vi "run.vi"(8 "error in (no error)":errorcluster, 11 "DL090409StageScaffold in":refnum<class "StageDL090409Scaffold.lvclass">) -> (0 "error out":errorcluster, 3 "DL090409StageScaffold out":refnum<class "StageDL090409Scaffold.lvclass">)   [LabVIEW 2010, in "StageDL090409Scaffold.lvclass"]
uses:
  StageDL090409Scaffold.lvclass
  main/labview_source/controls/undock_button.ctl
  internal_trigger_enum.ctl
  state_enum.ctl
  common/classes/SpaceVector/SpaceVector/SpaceVector.lvclass
  StageDL090409Scaffold.lvclass/StageDL090409Scaffold.ctl
  common/enumerations/top-level_component_type_enum.ctl
  GenericStage/GenericStage/trigger_enum.ctl
  GenericStage/GenericStage/translation_mode_enum.ctl
  stored_data_cluster.ctl
  common/classes/Image/Image/Image.lvclass
  Display/GenericDisplay/GenericDisplay/GenericDisplay.lvclass
  common/classes/GenericToplevelComponent/GenericToplevelComponent/trigger_type_enum.ctl
  GenericStage/GenericStage/GenericStage.lvclass
  common/classes/GenericToplevelComponent/GenericToplevelComponent/GenericToplevelComponent.lvclass
  common/classes/ErrorController/ErrorController/class_data.vi
  common/classes/ErrorController/ErrorController/ErrorController.lvclass
panel:
  in  "Tab Control":enum32{"User", "Debug", "About"}(tab)
  out "current x":dbl[unit] caption="x"
  out "current y":dbl[unit] caption="y"
  out "current z":dbl[unit] caption="z"
  in  "setOriginButton":bool
  in  "step x":dbl[unit] caption="x"
  in  "step y":dbl[unit] caption="y"
  in  "step z":dbl[unit] caption="z"
  in  "stepButton":bool
  in  "returnToOriginButton":bool
  in  "Stored positions":i32(listbox)
  in  "Description":string
  in  "store button":bool
  out "position image":T1(plugin-control)
  in  "go to stored button":bool
  in  "remove stored item":bool
  in  "step x 2":dbl[unit] caption="x"
  in  "step y 2":dbl[unit] caption="y"
  in  "step z 2":dbl[unit] caption="z"
  in  "moveAbsolute":bool
  in  "button:undock":T2
  out "finished?":bool
  out "last trigger":T3=enum."initialise"
  out "state":T4
  out "statemachine loop counter":i32
  out "event loop error":errorcluster
  out "statemachine error":errorcluster
  out "event loop counter":i32
  # "Move"
  # "Current position"
  # "Move To:"
  # "Make sure that\nALL axes have correct values!!!"
  # "StageDL090409Scaffold (or child class)\n\nimplemented by: Dominik Langer, University of Zurich\nmodified by: Marcel van 't Hoff, University of Zurich"
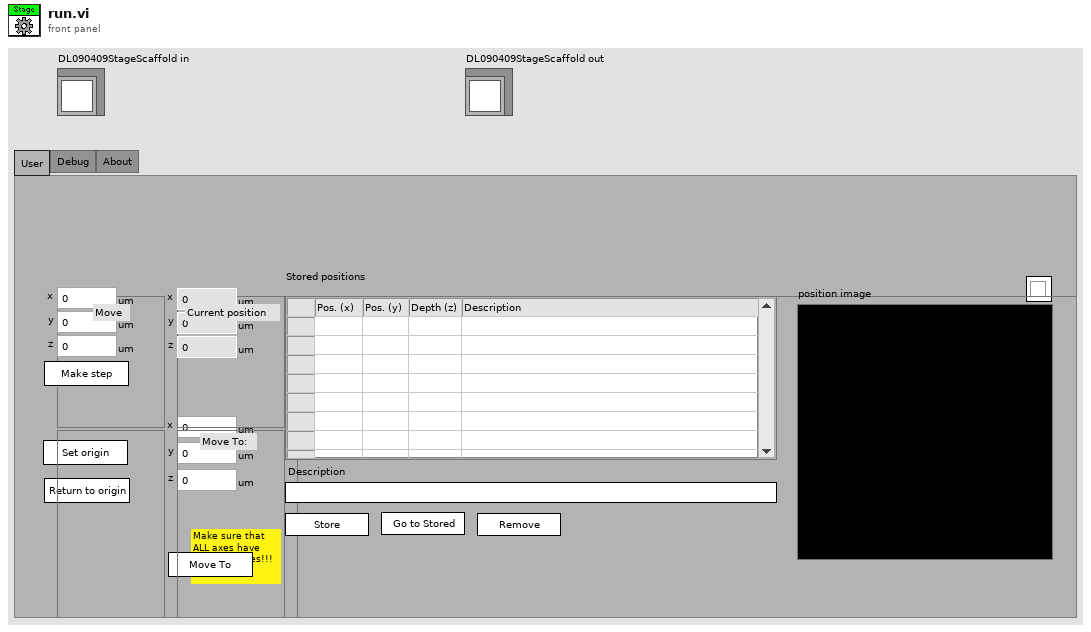
[diagram p1: front panel]
types:
  T1 = typedef "IMAQ Image.ctl" = refnum<image>
  T2 = typedef "undock_button.ctl" = bool
  T3 = typedef "StageDL090409Scaffold.lvclass/internal_trigger_enum.ctl" = enum16{"NULL", "initialise", "terminate", "move", "update position", "set origin", "return to origin", "attach observer", "detach observer", "go to stored"}
  T4 = typedef "StageDL090409Scaffold.lvclass/state_enum.ctl" = enum16{"idle", "moving"}
  T5 = typedef "top-level_component_type_enum.ctl" = enum16{"undefined", "ImagingMode", "ScanHead", "DAQ", "ImageAssembler", "Display", "DataCollection", "Analyser", "Stimulator", "ExperimentController", "Instrument", "Stage"}
  T6 = typedef "GenericStage.lvclass/trigger_enum.ctl" = enum16{"NULL", "move", "update position", "set origin", "return to origin"}
  T7 = typedef "GenericStage.lvclass/translation_mode_enum.ctl" = enum16{"DON'T MOVE", "relative", "absolute"}
  T8 = typedef "StageDL090409Scaffold.lvclass/stored_data_cluster.ctl" = cluster{"stored position":refnum<class "SpaceVector.lvclass">, "description":string, "position image":refnum<class "Image.lvclass">}
  T9 = typedef "trigger_type_enum.ctl" = enum8{"external", "internal", "common"}
  T10 = typedef "main_trigger_enum.ctl" = enum16{"NULL", "initialise", "terminate", "start", "stop", "change objective", "change experimentController", "change imagingMode", "save notebook", "started saving", "finished saving", "expCtr ready", "expCtr missing", "imgMd ready", "imgMd missing", "scanHd ready", "scanHd missing", "DAQ ready", "DAQ missing", "imgAsm ready", "imgAsm missing", "dataColl ready", "dataColl missing", "display ready", "display missing", "analysr ready", "analysr missing", "instrmnt ready", "instrmnt missing", "stimltr ready", "stimltr missing", "stage ready", "stage missing"}
  T11 = typedef "GenericToplevelComponent.lvclass/common_trigger_enum.ctl" = enum16{"NULL", "initialise", "terminate", "fetch command", "fetch data", "attach observer", "register as observer", "detach observer", "acknowledge", "start", "stop", "sweep started", "sweep finished", "experiment started", "experiment stopped"}
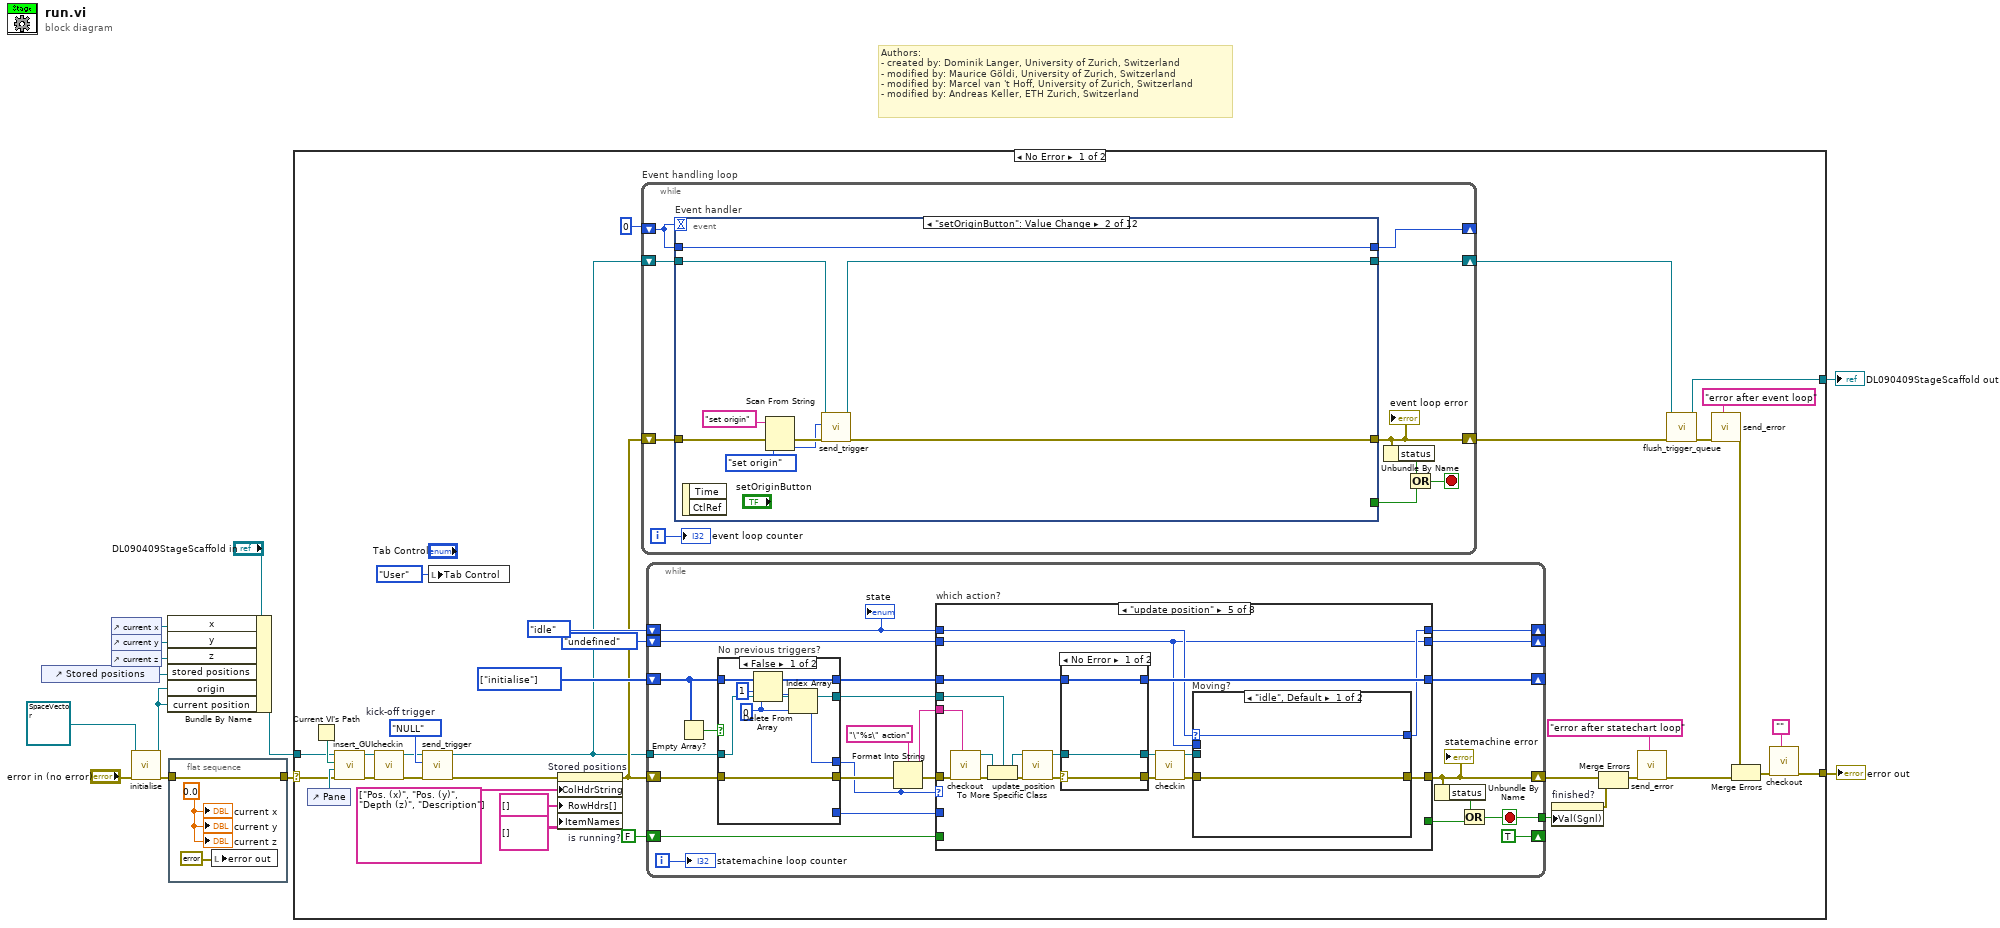
[diagram p0: block diagram]
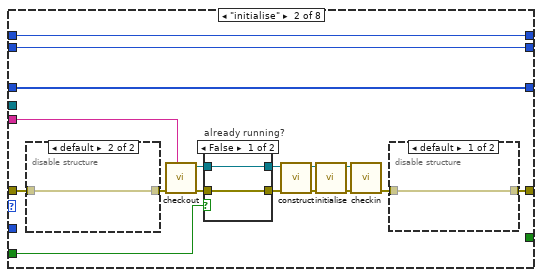
[diagram p3: hidden frame]
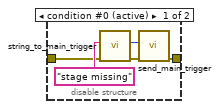
[diagram p4: hidden frame]
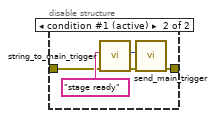
[diagram p5: hidden frame]
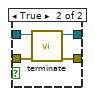
[diagram p6: hidden frame]
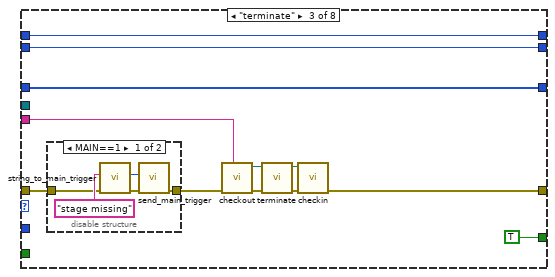
[diagram p7: hidden frame]
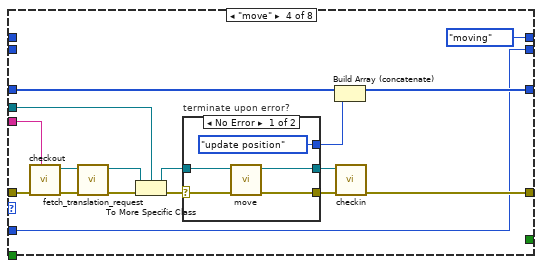
[diagram p9: hidden frame]
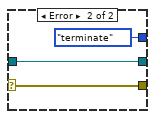
[diagram p10: hidden frame]
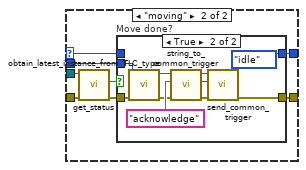
[diagram p11: hidden frame]
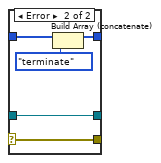
[diagram p13: hidden frame]
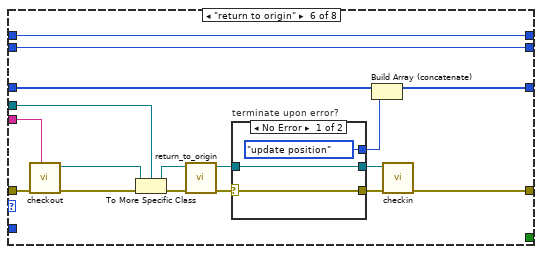
[diagram p14: hidden frame]
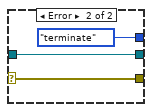
[diagram p15: hidden frame]
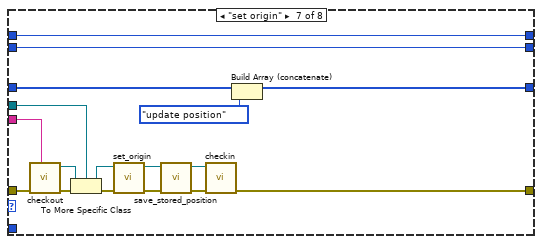
[diagram p16: hidden frame]
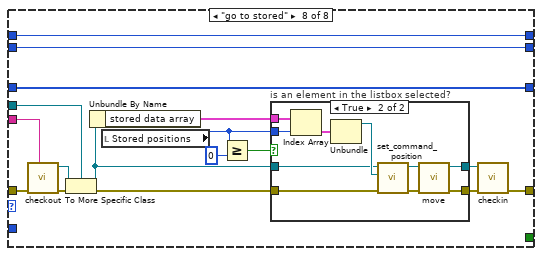
[diagram p17: hidden frame]
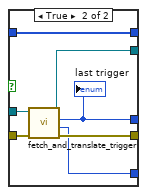
[diagram p19: hidden frame]
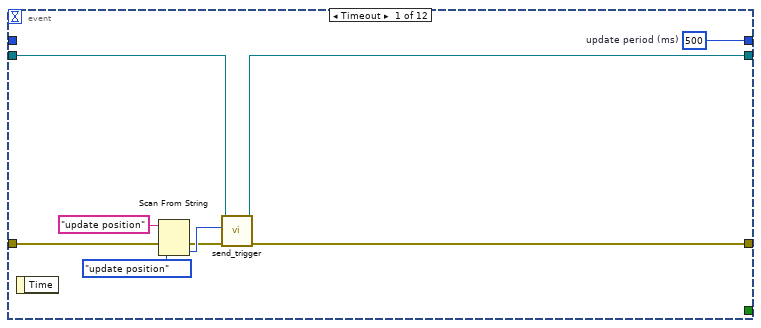
[diagram p20: hidden frame]
diagram:
  # "Authors: \n- created by: Dominik Langer, University of Zurich, Switzerland\n- modified by: Maurice Göldi, University of Zurich, Switzerland\n- modified by: Marcel van 't Hoff, University of Zurich, Switzerland\n- modified by: Andreas Keller, ETH Zurich, Switzerland"
  n1 = control-ref of="Stored positions"() -> (w6:refnum<vi>)
  n2 = control-ref of="current x"() -> (w9:refnum<vi>)
  n3 = control-ref of="current y"() -> (w8:refnum<vi>)
  n4 = control-ref of="current z"() -> (w7:refnum<vi>)
  n5 = call "initialise.vi"("error in (no error)"="error in (no error)", "SpaceVector in"=refnum<class "SpaceVector.lvclass"> refnum ("current position")) -> ("error out"=w2:errorcluster, "SpaceVector out"=w4:refnum<class "SpaceVector.lvclass">)  [unwired: 3 in, 5 out]
  n6 = Bundle By Name(cluster="DL090409StageScaffold in", "x"=w9, "y"=w8, "z"=w7, "stored positions"=w6, "origin"=w4, "current position"=w4) -> (w10:refnum<class "StageDL090409Scaffold.lvclass">)
  n7 = flat-sequence {
    tunnel: w2 -> [w15]
    tunnel: [w15] -> w1
    frame #0 {
      w16 = dbl[unit] 0.0 ("current x")
      n8 = local write "error out"(errorcluster {"status"=FALSE, "code"=0, "source"=""} ("error in (no error)")) -> ()
      "current x" <- w16
      "current y" <- w16
      "current z" <- w16
    }
  }
  n9 = case shown="No Error" w1 {
    selector: w1 -> [w44 w470]
    tunnel: [w50 w470] -> w13
    tunnel: [w31 w469] -> w12
    tunnel: w10 -> [w47 w469]
    frame No Error {
      w29 = FALSE  # is running?
      w30 = T3[] [enum."initialise"] items=["NULL", "initialise", "terminate", "move", "update position", "set origin", "return to origin", "attach observer", "detach observer", "go to stored"]
      w40 = trigger_enum."NULL"  # kick-off trigger
      n10 = control-ref of="Pane"() -> (w46:refnum<vi>)
      n11 = Current VI's Path() -> (path=w48:path)
      n12 = call-dynamic "insert_GUI.vi"("error in (no error)"=w44, "Pane"=w46, "VI path"=w48, "GenericComponent in"=w47) -> ("error out"=w22:errorcluster, "GenericComponent out"=w21:refnum<class "StageDL090409Scaffold.lvclass">)  [unwired: 6 in]
      n13 = call-dynamic "checkin.vi"("error in (no error)"=w22, "GenericStage in"=w21) -> ("error out"=w38:errorcluster, "GenericStage out"=w37:refnum<class "StageDL090409Scaffold.lvclass">)  [unwired: 8 in]
      n14 = call-dynamic "send_trigger.vi"("error in (no error)"=w38, "trigger"=w40, "GenericStage in"=w37) -> ("error out"=w41:errorcluster, "GenericStage out"=w19:refnum<class "StageDL090409Scaffold.lvclass">)  [unwired: 7 in]
      n15 = local write "Tab Control"(enum32{"User", "Debug", "About"}."User" ("Tab Control")) -> ()
      n16 = property on="Stored positions" class="MCListbox (strict)"(error in=w41, "ColHdrString"=string[] ["Pos. (x)", "Pos. (y)", "Depth (z)", "Description"] ("Row Header Strings[]"), "RowHdrs[]"=string[] [] ("Row Header Strings[]"), "ItemNames"=string[][] [] ("Item Names")) -> (error out=w20:errorcluster)  [unwired: 1 in, 1 out]
      n17 = while "Event handling loop" {
        shift-right: [w300] -> _
        shift-left: 0 -> [w301]
        shift-right: [w296] -> w33
        shift-left: w20 -> [w299]
        shift-right: [w297] -> w34
        shift-left: w19 -> [w298]
        i -> [w292]
        stop <- w293 stop-if-true
        n18 = event "Event handler" shown="[1] \"setOriginButton\": Value Change" {
          selector: _ -> [_ _ _ _ _ _ _ _ _ _ _ _]
          dyn-events: _ -> [_ _ _ _ _ _ _ _ _ _ _ _]
          timeout: w301 -> [_ _ _ _ _ _ _ _ _ _ _ _]
          tunnel: w301 -> [_ w319 w331 w343 w352 w384 w411 w425 w440 w447 w464 w468]
          tunnel: [w310 w319 w331 w343 w352 w384 w411 w425 w440 w447 w464 w468] -> w300
          tunnel: w299 -> [w303 w317 w330 w342 w346 w383 w406 w424 w433 w446 w463 w467]
          tunnel: [w307 w311 w324 w336 w349 w359 w405 w421 w427 w445 w459 w467] -> w296
          tunnel: [_ _ _ _ _ _ _ _ _ _ _ TRUE] -> w294
          tunnel: w298 -> [w309 w318 w323 w335 w351 w380 w410 w420 w429 w444 w456 w465]
          tunnel: [w308 w312 w321 w333 w350 w380 w410 w419 w429 w443 w455 w465] -> w297
          event Timeout {
            w310 = 500  # update period (ms)
            n19 = event-data() -> ()  [unwired: 2 out]
            n20 = Scan From String(input string="update position", error in=w303, default 1=trigger_enum."update position" ("trigger")) -> (error out=w302:errorcluster, output 1=w304:T6)  [unwired: 2 in, 2 out]
            n21 = call-dynamic "send_trigger.vi"("error in (no error)"=w302, "trigger"=w304, "GenericStage in"=w309) -> ("error out"=w307:errorcluster, "GenericStage out"=w308:refnum<class "StageDL090409Scaffold.lvclass">)  [unwired: 7 in]
          }
          event "setOriginButton": Value Change {
            n22 = event-data() -> ()  [unwired: 3 out]
            n23 = Scan From String(input string="set origin", error in=w317, default 1=trigger_enum."set origin" ("trigger")) -> (error out=w316:errorcluster, output 1=w313:T6)  [unwired: 2 in, 2 out]
            n24 = call-dynamic "send_trigger.vi"("error in (no error)"=w316, "trigger"=w313, "GenericStage in"=w318) -> ("error out"=w311:errorcluster, "GenericStage out"=w312:refnum<class "StageDL090409Scaffold.lvclass">)  [unwired: 7 in]
          }
          event "stepButton": Value Change {
            n25 = event-data() -> ()  [unwired: 3 out]
            n26 = call "initialise.vi"("z"="step z", "error in (no error)"=w330, "y"="step y", "x"="step x", "SpaceVector in"=refnum<class "SpaceVector.lvclass"> refnum ("current position")) -> ("error out"=w325:errorcluster, "SpaceVector out"=w326:refnum<class "SpaceVector.lvclass">)  [unwired: 5 in]
            n27 = call-dynamic "send_translation_request.vi"("error in (no error)"=w325, "translation mode"=translation_mode_enum."relative", "translation vector"=w326, "GenericStage in"=w323) -> ("error out"=w324:errorcluster, "GenericStage out"=w321:refnum<class "StageDL090409Scaffold.lvclass">)  [unwired: 6 in]
          }
          event "moveAbsolute": Value Change {
            # "Mirna: added this case 3/18/2015"
            n28 = event-data() -> ()  [unwired: 3 out]
            n29 = call "initialise.vi"("z"="step z 2", "error in (no error)"=w342, "y"="step y 2", "x"="step x 2", "SpaceVector in"=refnum<class "SpaceVector.lvclass"> refnum ("current position")) -> ("error out"=w337:errorcluster, "SpaceVector out"=w338:refnum<class "SpaceVector.lvclass">)  [unwired: 5 in]
            n30 = call-dynamic "send_translation_request.vi"("error in (no error)"=w337, "translation mode"=translation_mode_enum."absolute", "translation vector"=w338, "GenericStage in"=w335) -> ("error out"=w336:errorcluster, "GenericStage out"=w333:refnum<class "StageDL090409Scaffold.lvclass">)  [unwired: 6 in]
          }
          event "returnToOriginButton": Value Change {
            n31 = event-data() -> ()  [unwired: 3 out]
            n32 = Scan From String(input string="return to origin", error in=w346, default 1=trigger_enum."return to origin" ("trigger")) -> (error out=w345:errorcluster, output 1=w344:T6)  [unwired: 2 in, 2 out]
            n33 = call-dynamic "send_trigger.vi"("error in (no error)"=w345, "trigger"=w344, "GenericStage in"=w351) -> ("error out"=w349:errorcluster, "GenericStage out"=w350:refnum<class "StageDL090409Scaffold.lvclass">)  [unwired: 7 in]
          }
          event "store button": Value Change {
            n34 = event-data() -> ()  [unwired: 3 out]
            n35 = call "checkout.vi"("locked by?"="\"store button\": Value change", "error in (no error)"=w383) -> ("error out"=w382:errorcluster, "GenericStage out"=w381:refnum<class "GenericStage.lvclass">)  [unwired: 8 in]
            n36 = To More Specific Class(target class=w380, reference=w381, error in=w382) -> (specific class reference=w367:refnum<class "StageDL090409Scaffold.lvclass">, error out=w375:errorcluster)
            n37 = Unbundle By Name(w367) -> ("stored data array"=w369:T8[], "current position"=w372:refnum<class "SpaceVector.lvclass">)
            n38 = call "create.vi"("error in (no error)"=w375) -> ("error out"=w374:errorcluster, "Image out"=w373:refnum<class "Image.lvclass">)  [unwired: 9 in]
            n39 = disable-structure shown="DISPLAY==1" {
              disable-tunnel: w374 -> [w387 w390]
              disable-tunnel: [w386 w390] -> w364
              disable-tunnel: [w385 _] -> w362
              frame condition #0 (active) {
                n40 = call "obtain_latest_instance.vi"("error in (no error)"=w387) -> ("error out"=w389:errorcluster, "GenericDisplay out"=w388:refnum<class "GenericDisplay.lvclass">)  [unwired: 9 in]
                n41 = call-dynamic "get_current_RGB_image.vi"("error in (no error)"=w389, "GenericDisplay in"=w388) -> ("error out"=w386:errorcluster, "RGB image"=w385:refnum<class "Image.lvclass">)  [unwired: 7 in, 1 out]
              }
              frame condition #1 {
              }
            }
            n42 = call-dynamic "is_empty.vi"("error in (no error)"=w364, "Image in"=w362) -> ("error out"=w363:errorcluster, "emtpy?"=w360:bool, "Image out"=w361:refnum<class "Image.lvclass">)  [unwired: 7 in]
            n43 = case shown="False" w360 {
              tunnel: [w395 w397] -> w379
              tunnel: [w394 w396] -> w377
              tunnel: w373 -> [w393 w396]
              tunnel: w363 -> [w392 w397]
              tunnel: w361 -> [w391 _]
              frame False {
                n44 = call "copy.vi"("error in (no error)"=w392, "image to copy (source)"=w391, "Image in (target)"=w393) -> ("error out"=w395:errorcluster, "Image out"=w394:refnum<class "Image.lvclass">)  [unwired: 7 in]
              }
              frame True {
              }
            }
            n45 = call-dynamic "get_IMAQ_ref.vi"("error in (no error)"=w379, "Image.lvclass in"=w377) -> ("error out"=w358:errorcluster, "Image"=→"position image":T1, "Image.lvclass out"=w370:refnum<class "Image.lvclass">)  [unwired: 5 in, 2 out]
            n46 = Bundle(cluster=T8 {"stored position"=refnum, "description"="", "position image"=refnum} ("stored data"), "stored position"=w372, "description"="Description", "position image"=w370) -> (w368:T8)
            n47 = Build Array (concatenate)(w369, w368) -> (w365:T8[])
            n48 = Bundle By Name(cluster=w367, "stored data array"=w365) -> (w357:refnum<class "StageDL090409Scaffold.lvclass">)
            n49 = call-dynamic "list_stored_positions.vi"("error in (no error)"=w358, "StageDL090409Scaffold in"=w357) -> ("error out"=w356:errorcluster, "StageDL090409Scaffold out"=w355:refnum<class "StageDL090409Scaffold.lvclass">)  [unwired: 8 in]
            n50 = call-dynamic "save_stored_position.vi"("error in (no error)"=w356, "StageDL090409Scaffold in"=w355) -> ("error out"=w353:errorcluster, "StageDL090409Scaffold out"=w354:refnum<class "StageDL090409Scaffold.lvclass">)  [unwired: 8 in]
            n51 = call-dynamic "checkin.vi"("error in (no error)"=w353, "GenericStage in"=w354) -> ("error out"=w359:errorcluster)  [unwired: 8 in, 1 out]
          }
          event "remove stored item": Value Change {
            n52 = event-data() -> ()  [unwired: 3 out]
            n53 = call "checkout.vi"("locked by?"="\"remove item button\": Value change", "error in (no error)"=w406) -> ("error out"=w409:errorcluster, "GenericStage out"=w407:refnum<class "GenericStage.lvclass">)  [unwired: 8 in]
            n54 = To More Specific Class(target class=w410, reference=w407, error in=w409) -> (specific class reference=w403:refnum<class "StageDL090409Scaffold.lvclass">, error out=w404:errorcluster)
            n55 = in-place {
              n56 = in-place-cluster #1(w403) -> ("stored data array"=w413:T8[])
              n57 = local read "Stored positions"() -> (w414:i32)
              n58 = Delete From Array(array=w413, index=w414) -> (array with subset deleted=w412:T8[])  [unwired: 1 in, 1 out]
              n59 = in-place-cluster #1("stored data array"=w412) -> (w402:refnum<class "StageDL090409Scaffold.lvclass">)
            }
            n60 = call-dynamic "list_stored_positions.vi"("error in (no error)"=w404, "StageDL090409Scaffold in"=w402) -> ("error out"=w401:errorcluster, "StageDL090409Scaffold out"=w399:refnum<class "StageDL090409Scaffold.lvclass">)  [unwired: 8 in]
            n61 = call-dynamic "save_stored_position.vi"("error in (no error)"=w401, "StageDL090409Scaffold in"=w399) -> ("error out"=w400:errorcluster, "StageDL090409Scaffold out"=w398:refnum<class "StageDL090409Scaffold.lvclass">)  [unwired: 8 in]
            n62 = call-dynamic "checkin.vi"("error in (no error)"=w400, "GenericStage in"=w398) -> ("error out"=w405:errorcluster)  [unwired: 8 in, 1 out]
          }
          event "go to stored button": Value Change {
            n63 = event-data() -> ()  [unwired: 2 out]
            n64 = Scan From String(input string="go to stored", error in=w424, default 1=internal_trigger_enum."update position" ("internal trigger")) -> (error out=w422:errorcluster, output 1=w418:T3)  [unwired: 2 in, 2 out]
            n65 = To Variant(anything=w418) -> (Variant=w417:variant)
            n66 = call-dynamic "send_generic_trigger.vi"("error in (no error)"=w422, "trigger type"=trigger_type_enum."internal", "trigger variant"=w417, "GenericToplevelComponent in"=w420) -> ("error out"=w421:errorcluster, "GenericToplevelComponent out"=w419:refnum<class "StageDL090409Scaffold.lvclass">)  [unwired: 4 in, 2 out]
          }
          event "Stored positions": Mouse Up {
            n67 = event-data() -> ()  [unwired: 2 out]
            n68 = call "checkout.vi"("locked by?"="stored positions: Mouse Down", "error in (no error)"=w433) -> ("error out"=w434:errorcluster, "GenericStage out"=w430:refnum<class "GenericStage.lvclass">)  [unwired: 8 in]
            n69 = To More Specific Class(target class=w429, reference=w430, error in=w434) -> (specific class reference=w426:refnum<class "StageDL090409Scaffold.lvclass">, error out=w432:errorcluster)
            n70 = Unbundle By Name(w426) -> ("stored data array"=w439:T8[])
            n71 = Index Array(array=w439, index="Stored positions") -> (element=w438:T8)
            n72 = Unbundle By Name(w438) -> ("position image"=w437:refnum<class "Image.lvclass">)
            n73 = call-dynamic "get_IMAQ_ref.vi"("error in (no error)"=w432, "Image.lvclass in"=w437) -> ("error out"=w428:errorcluster, "Image"=w436:T1)  [unwired: 5 in, 3 out]
            n74 = local write "position image"(w436) -> ()
            n75 = call-dynamic "checkin.vi"("error in (no error)"=w428, "GenericStage in"=w426) -> ("error out"=w427:errorcluster)  [unwired: 8 in, 1 out]
          }
          event Value Change {
            n76 = event-data() -> ()  [unwired: 2 out]
            n77 = Current VI's Path() -> (path=w441:path)
            n78 = call-dynamic "undock.vi"("error in (no error)"=w446, "undock?"="button:undock", "VI path"=w441, "component in"=w444) -> ("error out"=w445:errorcluster, "component out"=w443:refnum<class "StageDL090409Scaffold.lvclass">)  [unwired: 6 in]
          }
          event "Stored positions": Edit Cell {
            n79 = event-data() -> ("Coords.Row"=w452:i32, "Coords.Column"=w454:i32, "String"=w453:string)  [unwired: 1 out]
            n80 = call "checkout.vi"("locked by?"="Stored position edited: Value Change", "error in (no error)"=w463) -> ("error out"=w460:errorcluster, "GenericStage out"=w461:refnum<class "GenericStage.lvclass">)  [unwired: 8 in]
            n81 = To More Specific Class(target class=w456, reference=w461, error in=w460) -> (specific class reference=w458:refnum<class "StageDL090409Scaffold.lvclass">, error out=w457:errorcluster)
            n82 = call-dynamic "change_stored_position.vi"("Row"=w452, "String"=w453, "Column"=w454, "error in (no error)"=w457, "specific class reference"=w458, "StageDL090409Scaffold in"=w456) -> ("error out"=w451:errorcluster, "specific class reference out"=w448:refnum<class "StageDL090409Scaffold.lvclass">, "StageDL090409Scaffold out"=w455:refnum<class "StageDL090409Scaffold.lvclass">)  [unwired: 3 in]
            n83 = call-dynamic "save_stored_position.vi"("error in (no error)"=w451, "StageDL090409Scaffold in"=w448) -> ("error out"=w449:errorcluster, "StageDL090409Scaffold out"=w450:refnum<class "StageDL090409Scaffold.lvclass">)  [unwired: 8 in]
            n84 = call-dynamic "checkin.vi"("error in (no error)"=w449, "GenericStage in"=w450) -> ("error out"=w459:errorcluster)  [unwired: 8 in, 1 out]
          }
          event "finished?": Value Change {
            n85 = event-data() -> ()  [unwired: 3 out]
          }
        }
        "event loop error" <- w296
        n86 = Unbundle By Name(w296) -> ("status"=w295:bool)
        n87 = Or(x=w295, y=w294) -> (x .or. y?=w293:bool)
        "event loop counter" <- w292
      }
      n88 = while {
        shift-right: [w61] -> w25
        shift-left: w20 -> [w76]
        shift-right: [w67] -> _
        shift-left: w30 -> [w73]
        shift-right: [TRUE ("is running?")] -> _
        shift-left: w29 -> [w64]
        tunnel: w19 -> [w75]
        tunnel: [w58] -> w28
        shift-right: [w56] -> _
        shift-left: state_enum."idle" ("state") -> [w57]
        shift-right: [w54] -> _
        shift-left: top-level_component_type_enum."undefined" ("sender TLC type") -> [w53]
        i -> [w55]
        stop <- w58 stop-if-true
        n89 = Empty Array?(array=w73) -> (empty?=w74:bool)
        n90 = case "No previous triggers?" shown="False" w74 {
          tunnel: w75 -> [w284 w288]
          tunnel: w76 -> [w282 w290]
          tunnel: [w284 w287] -> w68
          tunnel: [w280 w285] -> w70
          tunnel: [_ w286] -> w62
          tunnel: [w282 w289] -> w71
          tunnel: w73 -> [w283 w291]
          tunnel: [w279 w291] -> w66
          frame False {
            w277 = 0 ("index")
            n91 = Delete From Array(array=w283, length=1, index=w277) -> (deleted portion=w281:T3[], array with subset deleted=w279:T3[])
            n92 = Index Array(array=w281, index=w277) -> (element=w280:T3)
          }
          frame True {
            n93 = call-dynamic "fetch_and_translate_trigger.vi"("error in (no error)"=w290, "StageDL090409Scaffold in"=w288) -> ("error out"=w289:errorcluster, "sender TLC type"=w286:T5, "statechart trigger"=w285:T3, "StageDL090409Scaffold out"=w287:refnum<class "StageDL090409Scaffold.lvclass">)  [unwired: 6 in]
            "last trigger" <- w285
          }
        }
        n94 = Format Into String(format string="\"%s\" action", error in=w71, w70) -> (resulting string=w65:string, error out=w69:errorcluster)  [unwired: 1 in]
        n95 = case "which action?" shown="\"update position\"" w70 {
          tunnel: [w79 w86 w124 w141 w165 w219 w241 w250] -> w61
          tunnel: w69 -> [w79 w84 w117 w148 w176 w223 w245 w251]
          tunnel: w68 -> [_ _ _ w145 w175 w222 w242 w249]
          tunnel: [w80 w85 w127 w139 w169 w211 w239 w264] -> w67
          tunnel: w66 -> [w80 w85 w127 w140 w170 w210 w240 w264]
          tunnel: w65 -> [_ w91 w121 w149 w177 w224 w237 w248]
          tunnel: w64 -> [_ w92 _ _ _ _ _ _]
          tunnel: w62 -> [_ _ _ w134 _ _ _ _]
          tunnel: [_ _ TRUE _ _ _ _ _] -> w60
          tunnel: [w78 w82 w119 state_enum."moving" ("state") w164 w209 w236 w263] -> w56
          tunnel: w57 -> [w78 w82 w119 _ w161 w209 w236 w263]
          tunnel: [w77 w81 w118 w134 w159 w208 w235 w262] -> w54
          tunnel: w53 -> [w77 w81 w118 _ w159 w208 w235 w262]
          frame "NULL", Default {
          }
          frame "initialise" {
            n96 = disable-structure shown="default" {
              disable-tunnel: w84 -> [w99 w103]
              disable-tunnel: [w102 w103] -> w83
              frame condition #0 (active) {
                n97 = call "string_to_main_trigger.vi"("error in (no error)"=w99, "trigger string"="stage missing") -> ("error out"=w100:errorcluster, "main trigger"=w98:T10)  [unwired: 8 in]
                n98 = call "send_main_trigger.vi"("error in (no error)"=w100, "trigger"=w98) -> ("error out"=w102:errorcluster)  [unwired: 9 in]
              }
              frame condition #1 {
              }
            }
            n99 = call "checkout.vi"("locked by?"=w91, "error in (no error)"=w83) -> ("error out"=w93:errorcluster, "GenericStage out"=w90:refnum<class "GenericStage.lvclass">)  [unwired: 8 out]
            n100 = case "already running?" shown="False" w92 {
              tunnel: w93 -> [w110 w114]
              tunnel: w90 -> [w111 w115]
              tunnel: [w110 w113] -> w88
              tunnel: [w111 w112] -> w89
              frame False {
              }
              frame True {
                n101 = call-dynamic "terminate.vi"("error in (no error)"=w114, "GenericPlugin in"=w115) -> ("error out"=w113:errorcluster, "GenericPlugin out"=w112:refnum<class "GenericStage.lvclass">)  [unwired: 8 out]
              }
            }
            n102 = call-dynamic "construct.vi"("error in (no error)"=w88, "GenericPlugin in"=w89) -> ("error out"=w95:errorcluster, "GenericPlugin out"=w94:refnum<class "GenericStage.lvclass">)  [unwired: 2 in, 6 out]
            n103 = call-dynamic "initialise.vi"("error in (no error)"=w95, "GenericPlugin in"=w94) -> ("error out"=w96:errorcluster, "GenericPlugin out"=w97:refnum<class "GenericStage.lvclass">)  [unwired: 8 out]
            n104 = call-dynamic "checkin.vi"("error in (no error)"=w96, "GenericStage in"=w97) -> ("error out"=w87:errorcluster)  [unwired: 8 in, 1 out]
            n105 = disable-structure shown="default" {
              disable-tunnel: [w104 w109] -> w86
              disable-tunnel: w87 -> [w104 w107]
              frame condition #0 {
              }
              frame condition #1 (active) {
                n106 = call "string_to_main_trigger.vi"("error in (no error)"=w107, "trigger string"="stage ready") -> ("error out"=w106:errorcluster, "main trigger"=w105:T10)  [unwired: 8 in]
                n107 = call "send_main_trigger.vi"("error in (no error)"=w106, "trigger"=w105) -> ("error out"=w109:errorcluster)  [unwired: 9 in]
              }
            }
          }
          frame "terminate" {
            n108 = disable-structure shown="MAIN==1" {
              disable-tunnel: w117 -> [w129 w133]
              disable-tunnel: [w132 w133] -> w116
              frame condition #0 (active) {
                n109 = call "string_to_main_trigger.vi"("error in (no error)"=w129, "trigger string"="stage missing") -> ("error out"=w130:errorcluster, "main trigger"=w128:T10)  [unwired: 8 in]
                n110 = call "send_main_trigger.vi"("error in (no error)"=w130, "trigger"=w128) -> ("error out"=w132:errorcluster)  [unwired: 9 in]
              }
              frame condition #1 {
              }
            }
            n111 = call "checkout.vi"("locked by?"=w121, "error in (no error)"=w116) -> ("error out"=w125:errorcluster, "GenericStage out"=w123:refnum<class "GenericStage.lvclass">)  [unwired: 8 out]
            n112 = call-dynamic "terminate.vi"("error in (no error)"=w125, "GenericPlugin in"=w123) -> ("error out"=w126:errorcluster, "GenericPlugin out"=w122:refnum<class "GenericStage.lvclass">)  [unwired: 8 out]
            n113 = call-dynamic "checkin.vi"("error in (no error)"=w126, "GenericStage in"=w122) -> ("error out"=w124:errorcluster)  [unwired: 8 in, 1 out]
          }
          frame "move" {
            n114 = call "checkout.vi"("locked by?"=w149, "error in (no error)"=w148) -> ("error out"=w150:errorcluster, "GenericStage out"=w147:refnum<class "GenericStage.lvclass">)  [unwired: 8 out]
            n115 = call-dynamic "fetch_translation_request.vi"("error in (no error)"=w150, "GenericStage in"=w147) -> ("error out"=w146:errorcluster, "GenericStage out"=w144:refnum<class "GenericStage.lvclass">)  [unwired: 8 out]
            n116 = To More Specific Class(target class=w145, reference=w144, error in=w146) -> (specific class reference=w137:refnum<class "StageDL090409Scaffold.lvclass">, error out=w136:errorcluster)
            n117 = case "terminate upon error?" shown="No Error" w136 {
              selector: w136 -> [w154 w158]
              tunnel: w137 -> [w155 w157]
              tunnel: [w153 w157] -> w143
              tunnel: [w152 w158] -> w142
              tunnel: [internal_trigger_enum."update position" ("internal trigger enum") internal_trigger_enum."terminate" ("internal trigger enum")] -> w138
              frame No Error {
                n118 = call-dynamic "move.vi"("error in (no error)"=w154, "DL090409StageScaffold in"=w155) -> ("error out"=w152:errorcluster, "DL090409StageScaffold out"=w153:refnum<class "StageDL090409Scaffold.lvclass">)  [unwired: 8 out]
              }
              frame Error {
              }
            }
            n119 = Build Array (concatenate)(w140, w138) -> (w139:T3[])
            n120 = call-dynamic "checkin.vi"("error in (no error)"=w142, "GenericStage in"=w143) -> ("error out"=w141:errorcluster)  [unwired: 8 in, 1 out]
          }
          frame "update position" {
            n121 = call "checkout.vi"("locked by?"=w177, "error in (no error)"=w176) -> ("error out"=w167:errorcluster, "GenericStage out"=w168:refnum<class "GenericStage.lvclass">)  [unwired: 8 out]
            n122 = To More Specific Class(target class=w175, reference=w168, error in=w167) -> (specific class reference=w174:refnum<class "StageDL090409Scaffold.lvclass">, error out=w173:errorcluster)
            n123 = call-dynamic "update_position.vi"("error in (no error)"=w173, "DL090409StageScaffold in"=w174) -> ("error out"=w171:errorcluster, "DL090409StageScaffold out"=w172:refnum<class "StageDL090409Scaffold.lvclass">)  [unwired: 8 out]
            n124 = case shown="No Error" w171 {
              selector: w171 -> [w200 w207]
              tunnel: w172 -> [w201 w206]
              tunnel: [w201 w206] -> w163
              tunnel: [w200 w207] -> w162
              tunnel: w170 -> [w202 w205]
              tunnel: [w202 w204] -> w169
              frame No Error {
              }
              frame Error {
                n125 = Build Array (concatenate)(w205, internal_trigger_enum."terminate" ("internal trigger enum")) -> (w204:T3[])
              }
            }
            n126 = call-dynamic "checkin.vi"("error in (no error)"=w162, "GenericStage in"=w163) -> ("error out"=w166:errorcluster, "GenericStage out"=w160:refnum<class "StageDL090409Scaffold.lvclass">)  [unwired: 8 in]
            n127 = case "Moving?" shown="\"idle\", Default" w161 {
              selector: w161 -> [w178 w181]
              tunnel: w166 -> [w179 w185]
              tunnel: [w179 w187] -> w165
              tunnel: [w178 w180] -> w164
              tunnel: w160 -> [_ w186]
              tunnel: w159 -> [_ w183]
              frame "idle", Default {
              }
              frame "moving" {
                n128 = call-dynamic "get_status.vi"("error in (no error)"=w185, "StageDL090409Scaffold in"=w186) -> ("error out"=w184:errorcluster, "is happy?"=w182:bool)  [unwired: 7 in, 1 out]
                n129 = case "Move done?" shown="True" w182 {
                  tunnel: [w188 w199] -> w187
                  tunnel: w184 -> [w188 w198]
                  tunnel: w183 -> [_ w197]
                  tunnel: w181 -> [w189 _]
                  tunnel: [w189 state_enum."idle" ("state")] -> w180
                  frame False {
                  }
                  frame True {
                    n130 = call "obtain_latest_instance_from_TLC_type.vi"("error in (no error)"=w198, "top-level component type"=w197) -> ("error out"=w194:errorcluster, "GenericToplevelComponent.lvclass"=w190:refnum<class "GenericToplevelComponent.lvclass">)  [unwired: 8 in]
                    n131 = call-dynamic "string_to_common_trigger.vi"("error in (no error)"=w194, "trigger string"="acknowledge", "GenericToplevelComponent in"=w190) -> ("error out"=w193:errorcluster, "trigger"=w191:T11, "GenericToplevelComponent out"=w192:refnum<class "GenericToplevelComponent.lvclass">)  [unwired: 6 in]
                    n132 = call-dynamic "send_common_trigger.vi"("error in (no error)"=w193, "trigger"=w191, "GenericToplevelComponent in"=w192) -> ("error out"=w199:errorcluster)  [unwired: 6 in, 2 out]
                  }
                }
              }
            }
          }
          frame "return to origin" {
            n133 = call "checkout.vi"("locked by?"=w224, "error in (no error)"=w223) -> ("error out"=w217:errorcluster, "GenericStage out"=w218:refnum<class "GenericStage.lvclass">)  [unwired: 8 out]
            n134 = To More Specific Class(target class=w222, reference=w218, error in=w217) -> (specific class reference=w216:refnum<class "StageDL090409Scaffold.lvclass">, error out=w215:errorcluster)
            n135 = call-dynamic "return_to_origin.vi"("error in (no error)"=w215, "StageDL090409Scaffold in"=w216) -> ("error out"=w214:errorcluster, "StageDL090409Scaffold out"=w213:refnum<class "StageDL090409Scaffold.lvclass">)  [unwired: 8 in]
            n136 = case "terminate upon error?" shown="No Error" w214 {
              selector: w214 -> [w226 w230]
              tunnel: w213 -> [w227 w229]
              tunnel: [w227 w229] -> w221
              tunnel: [w226 w230] -> w220
              tunnel: [internal_trigger_enum."update position" ("internal trigger enum") internal_trigger_enum."terminate" ("internal trigger enum")] -> w212
              frame No Error {
              }
              frame Error {
              }
            }
            n137 = Build Array (concatenate)(w210, w212) -> (w211:T3[])
            n138 = call-dynamic "checkin.vi"("error in (no error)"=w220, "GenericStage in"=w221) -> ("error out"=w219:errorcluster)  [unwired: 8 in, 1 out]
          }
          frame "set origin" {
            n139 = call "checkout.vi"("locked by?"=w237, "error in (no error)"=w245) -> ("error out"=w244:errorcluster, "GenericStage out"=w246:refnum<class "GenericStage.lvclass">)  [unwired: 8 out]
            n140 = To More Specific Class(target class=w242, reference=w246, error in=w244) -> (specific class reference=w247:refnum<class "StageDL090409Scaffold.lvclass">, error out=w243:errorcluster)
            n141 = call-dynamic "set_origin.vi"("error in (no error)"=w243, "StageDL090409Scaffold in"=w247) -> ("error out"=w234:errorcluster, "StageDL090409Scaffold out"=w232:refnum<class "StageDL090409Scaffold.lvclass">)  [unwired: 8 in]
            n142 = call-dynamic "save_stored_position.vi"("error in (no error)"=w234, "StageDL090409Scaffold in"=w232) -> ("error out"=w233:errorcluster, "StageDL090409Scaffold out"=w231:refnum<class "StageDL090409Scaffold.lvclass">)  [unwired: 8 in]
            n143 = call-dynamic "checkin.vi"("error in (no error)"=w233, "GenericStage in"=w231) -> ("error out"=w241:errorcluster)  [unwired: 8 in, 1 out]
            n144 = Build Array (concatenate)(w240, internal_trigger_enum."update position" ("internal trigger enum")) -> (w239:T3[])
          }
          frame "go to stored" {
            n145 = call "checkout.vi"("locked by?"=w248, "error in (no error)"=w251) -> ("error out"=w256:errorcluster, "GenericStage out"=w258:refnum<class "GenericStage.lvclass">)  [unwired: 8 in]
            n146 = To More Specific Class(target class=w249, reference=w258, error in=w256) -> (specific class reference=w260:refnum<class "StageDL090409Scaffold.lvclass">, error out=w257:errorcluster)
            n147 = Unbundle By Name(w260) -> ("stored data array"=w252:T8[])
            n148 = local read "Stored positions"() -> (w254:i32)
            n149 = Greater Or Equal?(x=w254, y=0) -> (x >= y?=w253:bool)
            n150 = case "is an element in the listbox selected?" shown="True" w253 {
              tunnel: w252 -> [_ w276]
              tunnel: [w266 w272] -> w259
              tunnel: w257 -> [w266 w270]
              tunnel: w254 -> [_ w269]
              tunnel: w260 -> [w265 w268]
              tunnel: [w265 w267] -> w261
              frame False {
              }
              frame True {
                n151 = Index Array(array=w276, index=w269) -> (element=w275:T8)
                n152 = Unbundle(w275) -> ("stored position"=w274:refnum<class "SpaceVector.lvclass">)  [unwired: 2 out]
                n153 = call-dynamic "set_command_position.vi"("error in (no error)"=w270, "command position"=w274, "DL090409StageScaffold.lvclass in"=w268) -> ("error out"=w273:errorcluster, "DL090409StageScaffold.lvclass out"=w271:refnum<class "StageDL090409Scaffold.lvclass">)  [unwired: 7 in]
                n154 = call-dynamic "move.vi"("error in (no error)"=w273, "DL090409StageScaffold in"=w271) -> ("error out"=w272:errorcluster, "DL090409StageScaffold out"=w267:refnum<class "StageDL090409Scaffold.lvclass">)  [unwired: 8 in]
              }
            }
            n155 = call-dynamic "checkin.vi"("error in (no error)"=w259, "GenericStage in"=w261) -> ("error out"=w250:errorcluster)  [unwired: 8 in, 1 out]
          }
        }
        "statemachine error" <- w61
        n156 = Unbundle By Name(w61) -> ("status"=w59:bool)
        n157 = Or(x=w59, y=w60) -> (x .or. y?=w58:bool)
        "state" <- w57
        "statemachine loop counter" <- w55
      }
      n158 = property on="finished?" class="Bool (strict)"("Val(Sgnl)"=w28) -> (error out=w24:errorcluster)  [unwired: 2 in, 1 out]
      n159 = Merge Errors(w25, w24) -> (w23:errorcluster)
      n160 = call "send_error.vi"("additional message"="error after statechart loop", "error in (no error)"=w23) -> ("error out"=w42:errorcluster)  [unwired: 9 in]
      n161 = call-dynamic "flush_trigger_queue.vi"("error in (no error)"=w33, "GenericToplevelComponent in"=w34) -> ("error out"=w32:errorcluster, "GenericToplevelComponent out"=w31:refnum<class "StageDL090409Scaffold.lvclass">)  [unwired: 8 in]
      n162 = call "send_error.vi"("additional message"="error after event loop", "error in (no error)"=w32) -> ("error out"=w43:errorcluster)  [unwired: 9 in]
      n163 = Merge Errors(w43, w42) -> (w51:errorcluster)
      n164 = call "checkout.vi"("locked by?"="", "error in (no error)"=w51) -> ("error out"=w50:errorcluster)  [unwired: 8 in, 1 out]
    }
    frame Error {
    }
  }
  "error out" <- w13
  "DL090409StageScaffold out" <- w12
